vi "CheckEndOfByte.vi"(11 "Input":u32[](array[numeric])=array[4877 elements] format="%.0x") -> (0 "Cycle":u32, 1 "PID":u32, 2 "FeedBack":u32, 3 "SetPoint":u32, 4 "RemainingData":u32[](array[numeric]) format="%.0x", 5 "Plot?":bool)   [LabVIEW 2019]
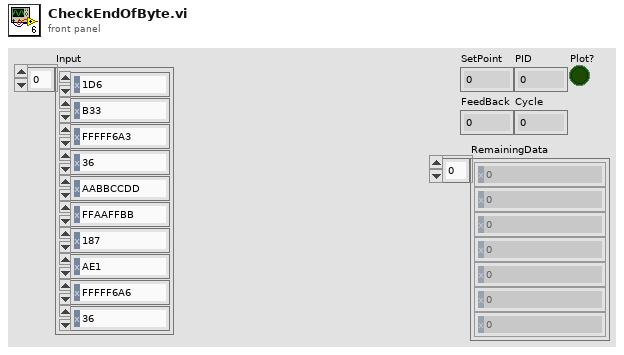
[diagram p1: front panel]
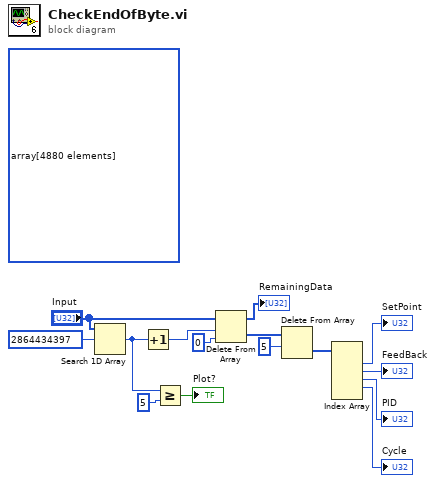
[diagram p0: block diagram]
diagram:
  (unwired) u32[] array[4880 elements] ("Array 2")
  n1 = Search 1D Array(1D array="Input", element=u32 2864434397 ("Output")) -> (index of element=w12:i32)  [unwired: 1 in]
  n2 = Increment(x=w12) -> (x+1=w9:i32)
  n3 = Greater Or Equal?(x=w12, y=5) -> (x >= y?=→"Plot?":bool)
  n4 = Delete From Array(array="Input", length=w9, index=0) -> (deleted portion=w8:u32[], array with subset deleted=→"RemainingData":u32[])
  n5 = Delete From Array(array=w8, length=5) -> (deleted portion=w6:u32[])  [unwired: 1 in, 1 out]
  n6 = Index Array(array=w6) -> (element #1=→"SetPoint":u32, element #2=→"FeedBack":u32, element #3=→"PID":u32, element #4=→"Cycle":u32)  [unwired: 5 in, 1 out]
